vi "Configure Arb Frequency [AF] Core.vi"(8 "error in (no error)":errorcluster, 9 "frequency (0.0 Hz)":dbl[unit] format="%.3f", 10 "channel name (\"CHANNEL1\")":string="CHANNEL1", 11 "IVI_Fgen in":refnum<class "IVI_Fgen.lvclass">) -> (0 "error out":errorcluster, 3 "IVI_Fgen out":refnum<class "IVI_Fgen.lvclass">)   [LabVIEW 2013, in "IVI_Fgen.lvlib" / "IVI_Fgen.lvclass"]
doc: "This VI configures the rate at which the function generator produces an entire cycle of an arbitrary waveform on a channel.\n \nNotes:\n\n(1) This VI is part of the IviFgenArbFrequency [AF] extension group."
uses:
  IVI_Fgen.lvclass
  IVI_Fgen.lvclass/IVI_Fgen.ctl
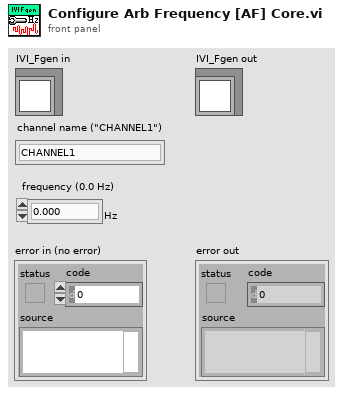
[diagram p1: front panel]
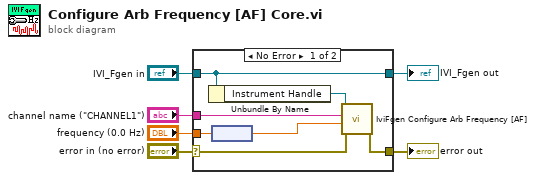
[diagram p0: block diagram]
diagram:
  n1 = case shown="No Error" "error in (no error)" {
    selector: "error in (no error)" -> [w11 w15]
    tunnel: [w10 w15] -> w5
    tunnel: [w13 w14] -> w3
    tunnel: "IVI_Fgen in" -> [w13 w14]
    tunnel: "frequency (0.0 Hz)" -> [w9 _]
    tunnel: "channel name (\"CHANNEL1\")" -> [w7 _]
    frame No Error {
      n2 = Unbundle By Name(w13) -> ("Instrument Handle"=w12:refnum<k15>)
      n3 = node(w9) -> (w8:dbl)
      n4 = call <vilib>:"IviFgen Configure Arb Frequency [AF].vi"("error in (no error)"=w11, "frequency (0.0 Hz)"=w8, "channel name (\"CHANNEL1\")"=w7, "instrument handle"=w12) -> ("error out"=w10:errorcluster)  [unwired: 6 in, 1 out]
    }
    frame Error {
    }
  }
  "error out" <- w5
  "IVI_Fgen out" <- w3
